vi "COBS Unstuff.vi"(8 "error in (no error)":errorcluster, 11 "Stuffed data in":u8[](array[numeric])) -> (0 "error out":errorcluster, 2 "Valid?":bool, 3 "Unstuffed Data":u8[](array[numeric]))   [LabVIEW 2015, in "LSR Transmission.lvlib"]
uses:
  LSR Transmission.lvlib
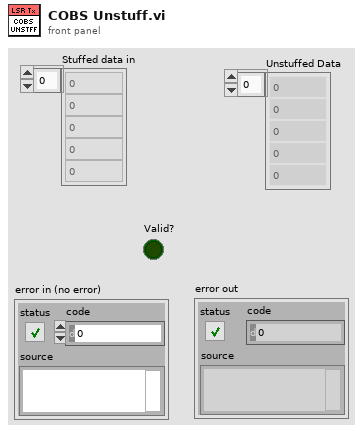
[diagram p1: front panel]
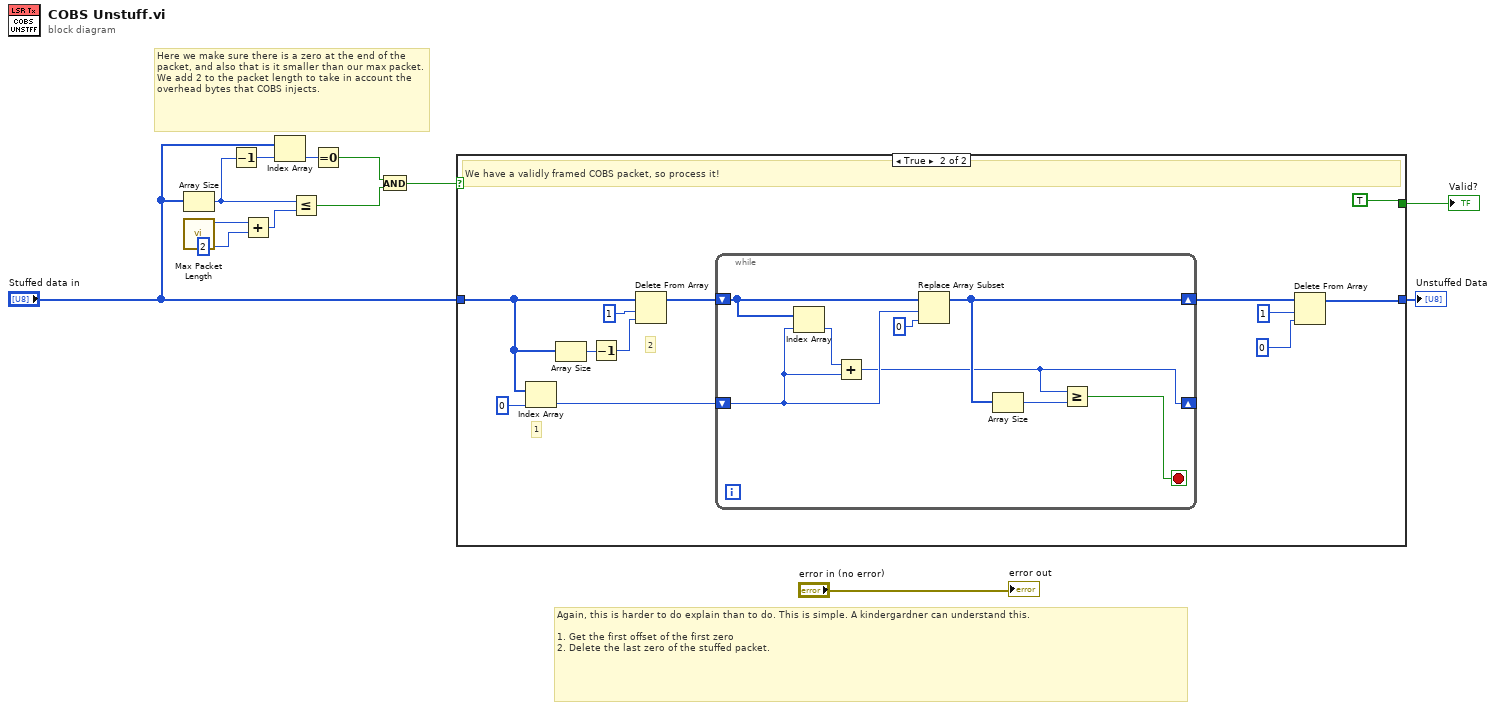
[diagram p0: block diagram]
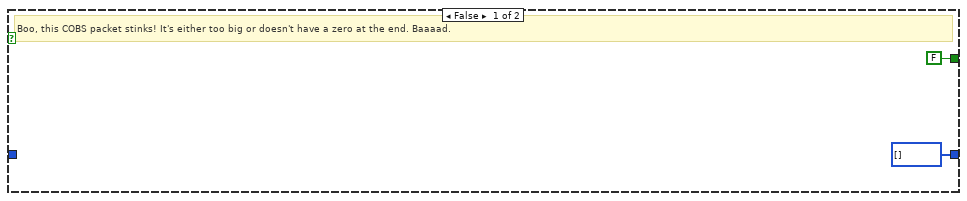
[diagram p2: hidden frame]
diagram:
  # "Here we make sure there is a zero at the end of the packet, and also that is it smaller than our max packet. We add 2 to the packet length to take in account the overhead bytes that COBS injects."
  # "Again, this is harder to do explain than to do. This is simple. A kindergardner can understand this. \n\n1. Get the first offset of the first zero\n2. Delete the last zero of the stuffed packet."
  n1 = Array Size(array="Stuffed data in") -> (size(s)=w10:i32)
  n2 = call "Max Packet Length.vi"() -> ("Max Packet Length"=w3:i32)  [unwired: 11 in]
  n3 = Decrement(x=w10) -> (x-1=w11:i32)
  n4 = Add(x=w3, y=2) -> (x+y=w2:i32)
  n5 = Index Array(array="Stuffed data in", index=w11) -> (element=w8:u8)
  n6 = Less Or Equal?(x=w10, y=w2) -> (x <= y?=w6:bool)
  n7 = Equal To 0?(x=w8) -> (x = 0?=w7:bool)
  n8 = And(x=w7, y=w6) -> (x .and. y?=w5:bool)
  n9 = case shown="True" w5 {
    tunnel: [u8[] [] ("Stuffed data in") w16] -> w4
    tunnel: "Stuffed data in" -> [_ w20]
    tunnel: [FALSE TRUE] -> w12
    frame False {
      # "Boo, this COBS packet stinks! It's either too big or doesn't have a zero at the end. Baaaad."
    }
    frame True {
      # "2"
      # "1"
      # "We have a validly framed COBS packet, so process it!"
      n10 = Index Array(array=w20, index=0) -> (element=w23:u8)
      n11 = Array Size(array=w20) -> (size(s)=w26:i32)
      n12 = Decrement(x=w26) -> (x-1=w27:i32)
      n13 = Delete From Array(array=w20, length=1, index=w27) -> (array with subset deleted=w24:u8[])  [unwired: 1 out]
      n14 = while {
        shift-right: [w29] -> _
        shift-left: w23 -> [w32]
        shift-right: [w31] -> w17
        shift-left: w24 -> [w35]
        stop <- w28 stop-if-true
        n15 = Index Array(array=w35, index=w32) -> (element=w33:u8)
        n16 = Add(x=w33, y=w32) -> (x+y=w29:u8)
        n17 = Replace Array Subset(array=w35, new element=u8 0 ("new element/subarray"), index=w32) -> (w31:u8[])
        n18 = Array Size(array=w31) -> (size(s)=w30:i32)
        n19 = Greater Or Equal?(x=w29, y=w30) -> (x >= y?=w28:bool)
      }
      n20 = Delete From Array(array=w17, length=1, index=0) -> (array with subset deleted=w16:u8[])  [unwired: 1 out]
    }
  }
  "Valid?" <- w12
  "Unstuffed Data" <- w4
  "error out" <- "error in (no error)"
